vi "LIN Init.vi"(9 "pConfig":T1, 10 "LINIndex":u8, 11 "DevHandle":i32) -> (3 "function return":i32)   [LabVIEW 2010, in "USB2XXX.lvlib"]
doc: "int WINAPI LIN_Init(int DevHandle,unsigned char LINIndex,LIN_CONFIG *pConfig);"
uses:
  USB2XXX.lvlib
  USB2XXX.dll
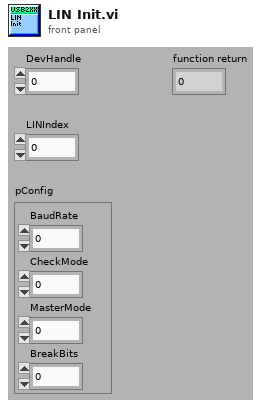
[diagram p1: front panel]
types:
  T1 = cluster{"BaudRate":u32, "CheckMode":u8, "MasterMode":u8, "BreakBits":u8}
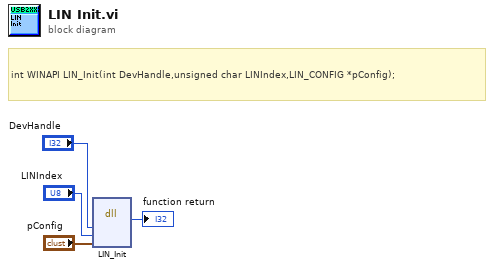
[diagram p0: block diagram]
diagram:
  # "int WINAPI LIN_Init(int DevHandle,unsigned char LINIndex,LIN_CONFIG *pConfig);"
  n1 = dll-call lib="F:/OtherWork/STM32/USB2XXX_Example/trunk/Labview/PublicFiles/USB2XXX.*" fn="LIN_Init"("DevHandle"="DevHandle", "LINIndex"="LINIndex", "pConfig"="pConfig") -> (→"function return":i32)  [unwired: 6 in, 2 out]
